vi "HIOKI PW3390 Conf Integ mode.vi"(0 "VISA Resource":refnum<visa-resource-name>, 1 "Set/Query (F: Set)":bool, 2 "CH (1)":i32=1 min=1 max=4, 5 "Mode (1: RMS)":enum16{"DC", "RMS"}(ring)=enum."RMS", 11 "error in (no error)":errorcluster, 12 "OPC query (T: ON)":bool=TRUE, 13 "Error Out (F: Off)":bool) -> (4 "VISA Resource out":refnum<visa-resource-name>, 6 "Mode out":enum16{"DC", "RMS"}(ring)=enum."RMS", 15 "error out":errorcluster)   [LabVIEW 2009]
doc: "Set/Query\n Set: Send the setting commands for the device.\n Query: Query the setting of the device.\n\nMode\n Sets the Integration Mode.\n\n<B>Note</B>\nDepending on the measurement line combination (for above 1P3W), the integration mode of other channels in the combination may be changed too."
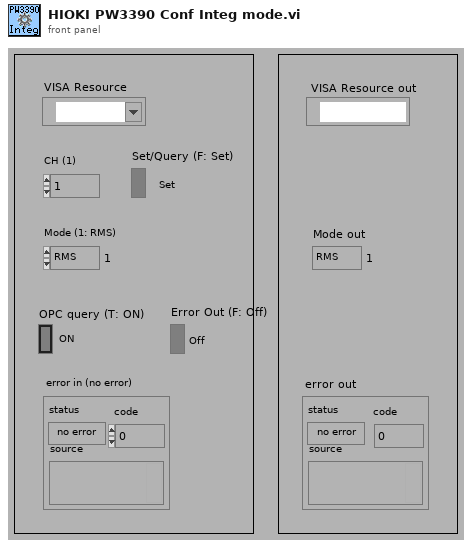
[diagram p1: front panel]
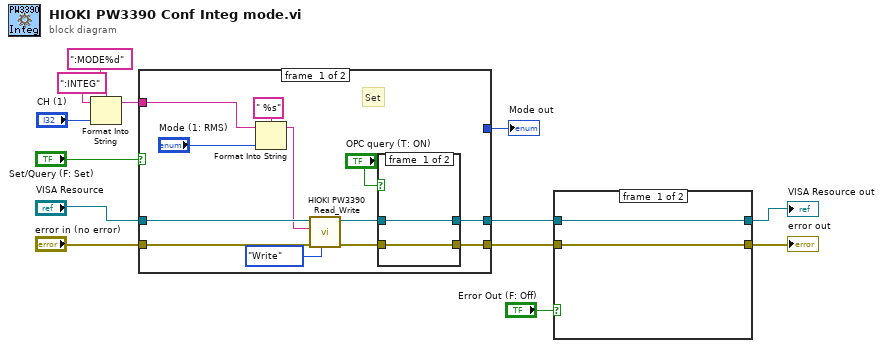
[diagram p0: block diagram]
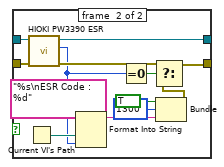
[diagram p2: hidden frame]
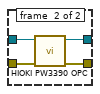
[diagram p3: hidden frame]
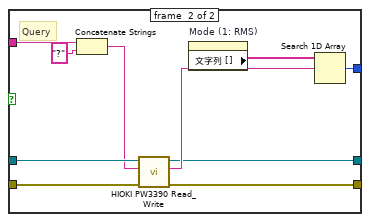
[diagram p4: hidden frame]
diagram:
  n1 = Format Into String(format string=":MODE%d", initial string=":INTEG", "CH (1)") -> (resulting string=w3:string)  [unwired: 1 in, 1 out]
  n2 = case shown="FALSE" "Set/Query (F: Set)" {
    tunnel: "error in (no error)" -> [w24 w40]
    tunnel: [w14 w33] -> w10
    tunnel: "VISA Resource" -> [w25 w41]
    tunnel: [w15 w32] -> w9
    tunnel: [_ w37] -> w7
    tunnel: w3 -> [w21 w36]
    frame #0 {
      # "Set"
      n3 = Format Into String(format string=" %s", initial string=w21, "Mode (1: RMS)") -> (resulting string=w19:string)  [unwired: 1 in, 1 out]
      n4 = call <instrlib>:"HIOKI PW3390 Read_Write.vi"("Read/Write"=enum16{"Read", "Write"}."Write", "error in (no error)"=w24, "data in"=w19, "VISA Resource"=w25) -> ("error out"=w16:errorcluster, "VISA Resource out"=w17:refnum<visa-resource-name>)  [unwired: 5 in, 1 out]
      n5 = case shown="TRUE" "OPC query (T: ON)" {
        tunnel: [w27 w31] -> w15
        tunnel: [w26 w30] -> w14
        tunnel: w17 -> [w27 w29]
        tunnel: w16 -> [w26 w28]
        frame #0 {
        }
        frame #1 {
          n6 = call <instrlib>:"HIOKI PW3390 OPC.vi"("error in (no error)"=w28, "VISA Resource"=w29) -> ("error out"=w30:errorcluster, "VISA Resource out"=w31:refnum<visa-resource-name>)  [unwired: 7 in, 1 out]
        }
      }
    }
    frame #1 {
      # "Query"
      n7 = Concatenate Strings(w36, "?" ("文字列")) -> (w35:string)
      n8 = call <instrlib>:"HIOKI PW3390 Read_Write.vi"("error in (no error)"=w40, "data in"=w35, "VISA Resource"=w41) -> ("error out"=w33:errorcluster, "data out"=w38:string, "VISA Resource out"=w32:refnum<visa-resource-name>)  [unwired: 6 in]
      n9 = property on="Mode (1: RMS)" class="Enum (strict)"() -> ("文字列 []"=w39:string[])  [unwired: 2 in, 2 out]
      n10 = Search 1D Array(1D array=w39, element=w38) -> (index of element=w37:i32)  [unwired: 1 in]
    }
  }
  "Mode out" <- w7
  n11 = case shown="TRUE" "Error Out (F: Off)" {
    tunnel: w9 -> [w43 w56]
    tunnel: w10 -> [w42 w55]
    tunnel: [w42 w45] -> w8
    tunnel: [w43 w54] -> w1
    frame #0 {
    }
    frame #1 {
      n12 = Current VI's Path() -> (path=w52:path)
      n13 = call <instrlib>:"HIOKI PW3390 ESR.vi"("error in (no error)"=w55, "VISA Resource"=w56) -> ("error out"=w46:errorcluster, "Output Value"=w44:u8, "VISA Resource out"=w54:refnum<visa-resource-name>)  [unwired: 6 in, 1 out]
      n14 = Format Into String(format string="%s\nESR Code : %d", w52, w44) -> (resulting string=w48:string)  [unwired: 2 in, 1 out]
      n15 = Equal To 0?(x=w44) -> (x = 0?=w53:bool)
      n16 = Bundle("status"=TRUE, "code"=1300, w48) -> (w47:cluster{"status":bool, "code":i32, string})  [unwired: 1 in]
      n17 = Select(t=w46, s=w53, f=w47) -> (s? t:f=w45:errorcluster)
    }
  }
  "error out" <- w8
  "VISA Resource out" <- w1
